vi "Autonomous Independent.vi"   [LabVIEW 2013]
doc: "This VI is called when autonomous begins, and will automatically be terminated when autonomous ends. You can carry out timed or sensor driven robot movement independently without needing to return to the caller."
uses:
  <vilib>/Rock Robotics/WPI/Solenoid/WPI_SolenoidValue.ctl
  Robot Global Data.vi
  <vilib>/Rock Robotics/WPI/RobotDrive/WPI_RobotDriveGetSetRefNum.vi
  <vilib>/Rock Robotics/WPI/RobotDrive/WPI_RobotDriveArcadeDrive_Standard(NoSaturation).vi
  <vilib>/Rock Robotics/WPI/Solenoid/Deprecated/WPI_SolenoidGetBool.vi
  <vilib>/Rock Robotics/WPI/Solenoid/WPI_SolenoidSetEnum.vi
  <vilib>/Rock Robotics/WPI/Joystick/WPI_JoystickGetSetRefNum.vi
panel:
  # "Be sure to right-click and choose Data Operations>>Make Current Value default if you want to save the array values with the VI"
types:
  T1 = typedef "WPI_SolenoidDevRef.ctl" = cluster{"DevStatus":errorcluster, "Solenoid Module":T2, "Forward Solenoid Channel":T3, "Reverse Solenoid Channel":T3}
  T2 = typedef "FPGA_TypedefSolenoidModule.ctl" = enum16{"Solenoid Module 1", "Solenoid Module 2"}
  T3 = typedef "WPI_SolenoidChannel.ctl" = enum8{"Solenoid 1", "Solenoid 2", "Solenoid 3", "Solenoid 4", "Solenoid 5", "Solenoid 6", "Solenoid 7", "Solenoid 8", "Invalid"}
  T4 = typedef "WPI_MotorControlDeviceRef.ctl" = cluster{"DeviceStatus":errorcluster, "Type":enum16{"PWM", "CAN"}, "PWM":cluster{"Digital Module":T5, "PWM Channel":T6, "DeadBand":T7}, "CAN":cluster{"Device Number":u8, "Control Mode":T8, "Semaphore":T9, "Max Vout":dbl}, "Invert":bool, "TransformRef":T10, "InvTransformRef":T10}
  T5 = typedef "FPGA_TypedefDigitalModule.ctl" = enum16{"Digital Module 1", "Digital Module 2"}
  T6 = typedef "FPGA_DIOPWMChannel.ctl" = enum8{"PWM 1", "PWM 2", "PWM 3", "PWM 4", "PWM 5", "PWM 6", "PWM 7", "PWM 8", "PWM 9", "PWM 10", "Invalid"}
  T7 = typedef "WPI_PWMDeadband.ctl" = cluster{"Name":string, "maxPositivePwm":i32, "minPositivePwm":i32, "centerPwm":i32, "maxNegativePwm":i32, "minNegativePwm":i32, "angularRange":u16}
  T8 = typedef "WPI_CANJaguar_ControlMode.ctl" = enum8{"Percent VBus", "Current", "Speed", "Position", "Voltage"}
  T9 = typedef "Semaphore RefNum" = refnum<k1>
  T10 = typedef "WPI_PWMTransform_ConPane.ctl" = refnum<vi>
  T11 = typedef "WPI_RobotDriveDevRef.ctl" = cluster{"DevStatus":errorcluster, "Motors[]":T4[], "Square Inputs":bool, "Max Output":dbl, "Isochronous":bool}
  T12 = typedef "WPI_JoystickDevRef.ctl" = cluster{"Device":T13}
  T13 = typedef "WPI_JoystickDeviceEnum.ctl" = enum16{"USB 1", "USB 2", "USB 3", "USB 4", "Kinect 1", "Kinect 2"}
  T14 = typedef "WPI_SolenoidValue.ctl" = enum16{"Off", "On", "Forward", "Reverse"}
  T15 = cluster{"axis 1 (x)":dbl, "axis 2 (y)":dbl, "axis 3 (throttle)":dbl, "axis 4":dbl, "axis 5":dbl, "axis 6":dbl}
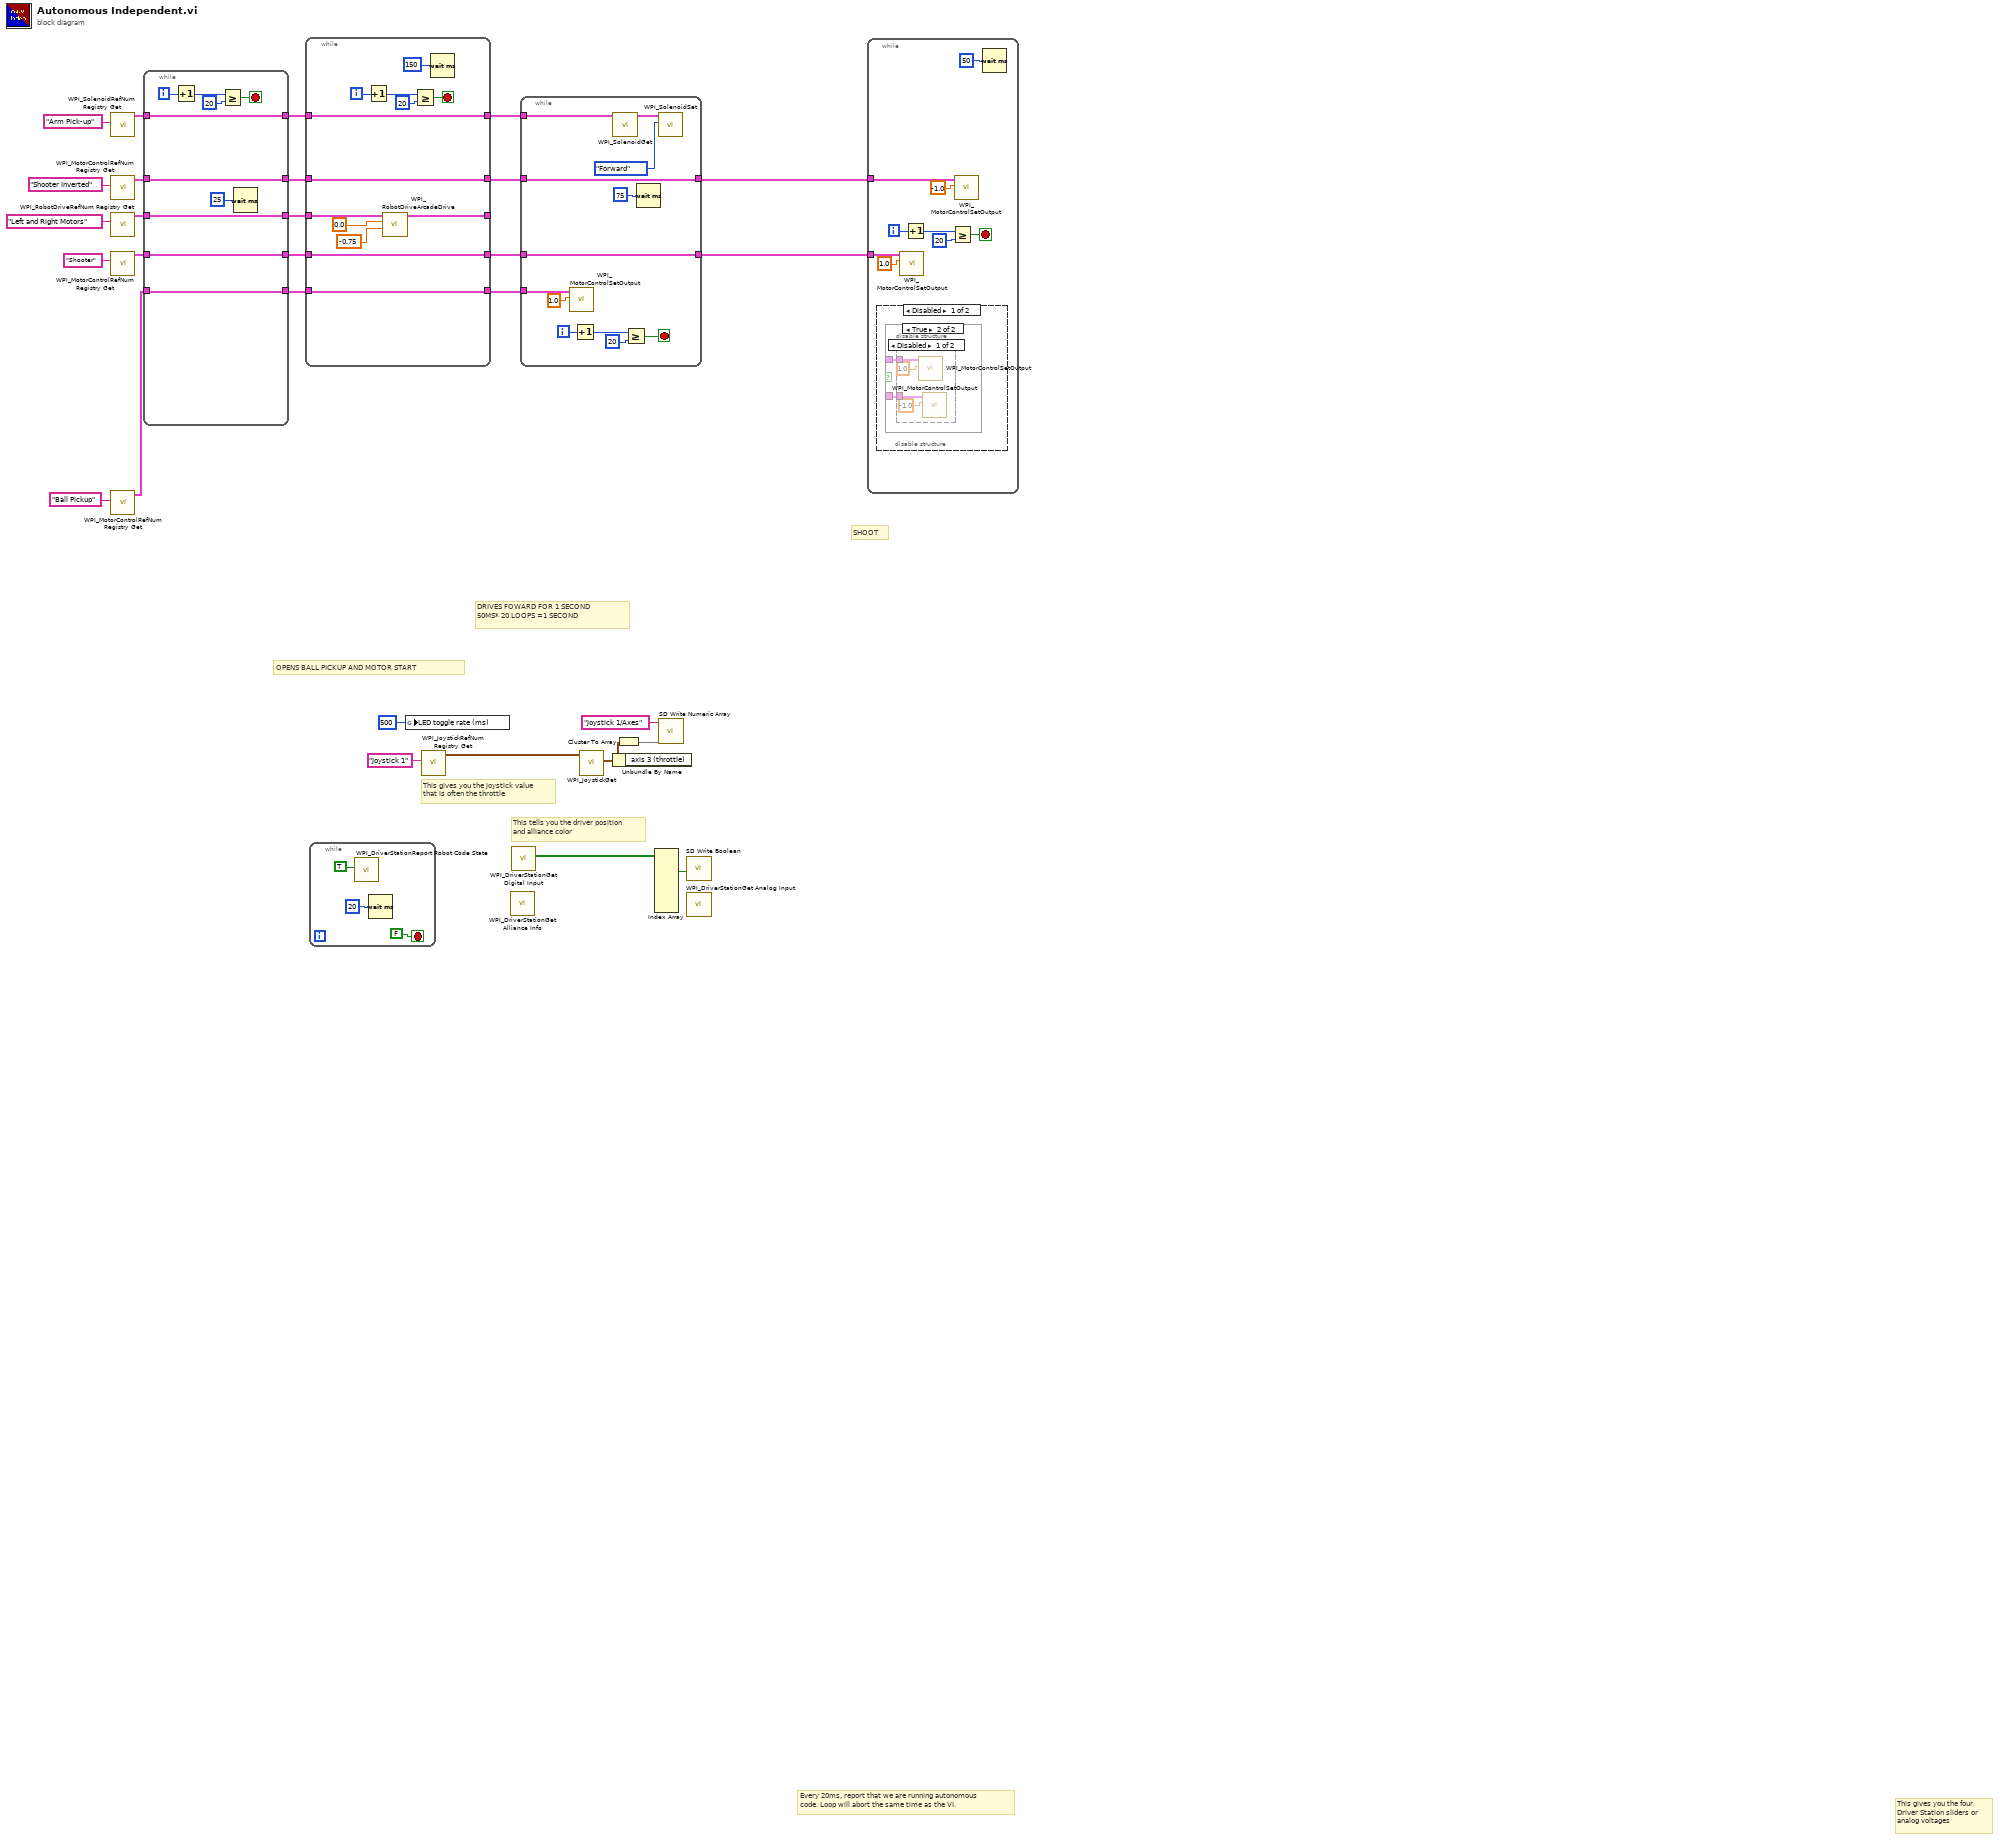
[diagram p0: block diagram]
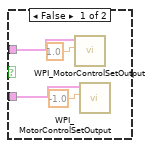
[diagram p2: hidden frame]
diagram:
  # "SHOOT"
  # "OPENS BALL PICKUP AND MOTOR START"
  # "DRIVES FOWARD FOR 1 SECOND\n50MS* 20 LOOPS =1 SECOND"
  # "Every 20ms, report that we are running autonomous\ncode. Loop will abort the same time as the VI."
  # "This gives you the joystick value\nthat is often the throttle"
  # "This tells you the driver position\nand alliance color"
  # "This gives you the four\nDriver Station sliders or\nanalog voltages"
  n1 = call <vilib>:"WPI_SolenoidRefNum Registry Get.vi"("refnum name"="Arm Pick-up") -> ("SolenoidDevRef"=w19:T1)  [unwired: 9 in, 1 out]
  n2 = call <vilib>:"WPI_MotorControlRefNum Registry Get.vi"("refnum name"="Shooter Inverted") -> ("MotorControlDevRef"=w15:T4)  [unwired: 9 in, 1 out]
  n3 = call <vilib>:"WPI_RobotDriveRefNum Registry Get.vi"("refnum name"="Left and Right Motors") -> ("RobotDriveDevRef"=w18:T11)  [unwired: 9 in, 1 out]
  n4 = call <vilib>:"WPI_MotorControlRefNum Registry Get.vi"("refnum name"="Shooter") -> ("MotorControlDevRef"=w14:T4)  [unwired: 9 in, 1 out]
  n5 = call <vilib>:"WPI_MotorControlRefNum Registry Get.vi"("refnum name"="Ball Pickup") -> ("MotorControlDevRef"=w12:T4)  [unwired: 9 in, 1 out]
  n6 = while {
    tunnel: w19 -> [w31]
    tunnel: [w39] -> w11
    tunnel: w18 -> [w39]
    tunnel: w15 -> [w33]
    tunnel: [w33] -> w9
    tunnel: w14 -> [w32]
    tunnel: [w32] -> w10
    tunnel: w12 -> [w30]
    tunnel: [w31] -> w4
    tunnel: [w30] -> w2
    i -> [w36]
    stop <- w35 stop-if-true
    n7 = Increment(x=w36) -> (x+1=w37:i32)
    n8 = Greater Or Equal?(x=w37, y=20) -> (x >= y?=w35:bool)
    n9 = Wait (ms)(milliseconds to wait=u32 25) -> ()  [unwired: 1 out]
  }
  n10 = while {
    tunnel: w11 -> [w52]
    tunnel: [w45] -> _
    tunnel: w9 -> [w43]
    tunnel: [w43] -> w7
    tunnel: w10 -> [w42]
    tunnel: [w42] -> w5
    tunnel: w4 -> [w41]
    tunnel: [w41] -> w3
    tunnel: [w40] -> w1
    tunnel: w2 -> [w40]
    i -> [w50]
    stop <- w47 stop-if-true
    n11 = Increment(x=w50) -> (x+1=w49:i32)
    n12 = call-poly <vilib>:"WPI_RobotDriveArcadeDrive.vi"("Y axis value"=-0.75, "X axis value"=0.0, "RobotDriveDevRef"=w52) -> ("RobotDriveDevRef"=w45:T11)  [unwired: 6 in, 2 out]
    n13 = Greater Or Equal?(x=w49, y=20) -> (x >= y?=w47:bool)
    n14 = Wait (ms)(milliseconds to wait=u32 150) -> ()  [unwired: 1 out]
  }
  n15 = while {
    stop <- FALSE stop-if-true
    n16 = call <vilib>:"WPI_DriverStationReport Robot Code State.vi"("Autonomous"=TRUE) -> ()  [unwired: 10 in, 1 out]
    n17 = Wait (ms)(milliseconds to wait=u32 20) -> ()  [unwired: 1 out]
  }
  n18 = global write "Robot Global Data.vi" "LED toggle rate (ms)"(u32 500 ("LED ms toggle rate")) -> ()
  n19 = call <vilib>:"WPI_JoystickRefNum Registry Get.vi"("refnum name"="Joystick 1") -> ("JoystickDevRef"=w27:T12)  [unwired: 1 in, 9 out]
  n20 = call <vilib>:"WPI_DriverStationGet Alliance Info.vi"() -> ()  [unwired: 12 out]
  n21 = call <vilib>:"WPI_DriverStationGet Digital Input.vi"() -> ("Driver Station Digital Input (1-8)"=w29:bool[])  [unwired: 11 out]
  n22 = while {
    tunnel: [w67] -> w8
    tunnel: w7 -> [w67]
    tunnel: [w66] -> w6
    tunnel: w5 -> [w66]
    tunnel: w3 -> [w58]
    tunnel: w1 -> [w56]
    i -> [w64]
    stop <- w62 stop-if-true
    n23 = call <vilib>:"WPI_MotorControlSetOutput.vi"("Output"=1.0, "MotorControlDevRef"=w56) -> ()  [unwired: 7 in, 3 out]
    n24 = Increment(x=w64) -> (x+1=w65:i32)
    n25 = call-poly <vilib>:"WPI_SolenoidGet.vi"("SolenoidDevRef"=w58) -> ("SolenoidDevRef"=w59:T1)  [unwired: 8 in, 2 out]
    n26 = Greater Or Equal?(x=w65, y=20) -> (x >= y?=w62:bool)
    n27 = Wait (ms)(milliseconds to wait=u32 75) -> ()  [unwired: 1 out]
    n28 = call-poly <vilib>:"WPI_SolenoidSet.vi"("Value"=WPI_SolenoidValue."Forward", "SolenoidDevRef"=w59) -> ()  [unwired: 8 in, 2 out]
  }
  n29 = call <vilib>:"WPI_JoystickGet.vi"("JoystickDevRef"=w27) -> ("Axes"=w24:T15)  [unwired: 1 in, 5 out]
  n30 = Unbundle By Name(w24) -> ()  [unwired: 1 out]
  n31 = Cluster To Array(cluster=w24) -> (array=w25:dbl[])
  n32 = Index Array(array=w29) -> (element #2=w22:bool)  [unwired: 8 in, 7 out]
  n33 = call <vilib>:"SD Write Numeric Array.vi"("Numeric Array"=w25, "Name"="Joystick 1/Axes") -> ()  [unwired: 8 in, 2 out]
  n34 = call <vilib>:"SD Write Boolean.vi"("Boolean"=w22) -> ()  [unwired: 9 in, 2 out]
  n35 = call <vilib>:"WPI_DriverStationGet Analog Input.vi"() -> ()  [unwired: 12 out]
  n36 = while {
    tunnel: w8 -> [w71]
    tunnel: w6 -> [w70]
    i -> [w74]
    stop <- w73 stop-if-true
    n37 = disable-structure shown="Disabled" {
      frame Disabled {
        n38 = case shown="True" {
          selector: _ -> [_ _]
          tunnel: _ -> [w78 w82]
          tunnel: _ -> [w77 w81]
          frame False {
            n39 = call <vilib>:"WPI_MotorControlSetOutput.vi"("Output"=1.0, "MotorControlDevRef"=w78) -> ()  [unwired: 7 in, 3 out]
            n40 = call <vilib>:"WPI_MotorControlSetOutput.vi"("Output"=-1.0, "MotorControlDevRef"=w77) -> ()  [unwired: 7 in, 3 out]
          }
          frame True {
            n41 = disable-structure shown="Disabled" {
              disable-tunnel: w82 -> [w86 _]
              disable-tunnel: w81 -> [w83 _]
              frame Disabled {
                n42 = call <vilib>:"WPI_MotorControlSetOutput.vi"("Output"=1.0, "MotorControlDevRef"=w86) -> ()  [unwired: 7 in, 3 out]
                n43 = call <vilib>:"WPI_MotorControlSetOutput.vi"("Output"=-1.0, "MotorControlDevRef"=w83) -> ()  [unwired: 7 in, 3 out]
              }
              frame Enabled {
              }
            }
          }
        }
      }
      frame Enabled {
      }
    }
    n44 = call <vilib>:"WPI_MotorControlSetOutput.vi"("Output"=1.0, "MotorControlDevRef"=w70) -> ()  [unwired: 7 in, 3 out]
    n45 = Increment(x=w74) -> (x+1=w76:i32)
    n46 = Greater Or Equal?(x=w76, y=20) -> (x >= y?=w73:bool)
    n47 = call <vilib>:"WPI_MotorControlSetOutput.vi"("Output"=-1.0, "MotorControlDevRef"=w71) -> ()  [unwired: 7 in, 3 out]
    n48 = Wait (ms)(milliseconds to wait=u32 50) -> ()  [unwired: 1 out]
  }
